vi "Check array is unique.vi"(10 "'Hold' list":bool[][](array[boolean]), 11 "Coins State Cache":bool[](array[boolean])) -> (3 "Is unique?":bool)   [LabVIEW 2014]
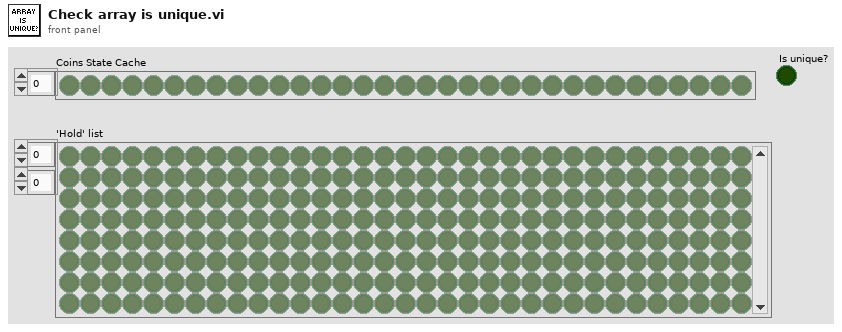
[diagram p1: front panel]
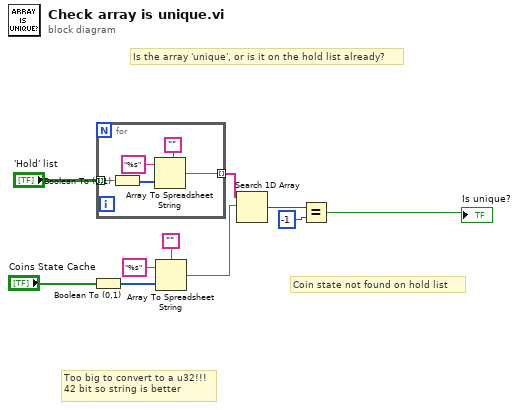
[diagram p0: block diagram]
diagram:
  # "Is the array 'unique', or is it on the hold list already?"
  # "Coin state not found on hold list"
  # "Too big to convert to a u32!!!\n42 bit so string is better"
  n1 = Boolean To (0,1)(Boolean="Coins State Cache") -> (0, 1=w1:i16[])
  n2 = for {
    tunnel: "'Hold' list" -> [w14] mode=indexing
    tunnel: [w12] -> w5 mode=indexing
    n3 = Boolean To (0,1)(Boolean=w14) -> (0, 1=w13:i16[])
    n4 = Array To Spreadsheet String(delimiter (Tab)="", array=w13, 3:"%s" ("format string")) -> (spreadsheet string=w12:string)
  }
  n5 = Array To Spreadsheet String(delimiter (Tab)="", array=w1, 3:"%s" ("format string")) -> (spreadsheet string=w3:string)
  n6 = Search 1D Array(1D array=w5, element=w3) -> (index of element=w7:i32)  [unwired: 1 in]
  n7 = Equal?(x=w7, y=-1) -> (x = y?=→"Is unique?":bool)
